vi "setup.vi"(8 "error in (no error)":errorcluster) -> (0 "error out":errorcluster, 3 "DAQmx_pulse_out out":refnum<class "DAQmx_pulse_out.lvclass">)   [LabVIEW 2013, in "DAQmx_pulse_out.lvclass"]
uses:
  DAQmx_pulse_out.lvclass
  DAQmx_pulse_out.lvclass/DAQmx_pulse_out.ctl
  <vilib>/DAQmx/write.llb/DAQmx Write (Digital 1D U8 1Chan NSamp).vi
  Globals.vi
  <vilib>/DAQmx/create/channels.llb/DAQmx Create Channel (DO-Digital Output).vi
  <vilib>/DAQmx/configure/timing.llb/DAQmx Timing (Sample Clock).vi
  <vilib>/DAQmx/configure/trigger.llb/DAQmx Start Trigger (Digital Edge).vi
  <vilib>/DAQmx/miscellaneous.llb/DAQmx Fill In Error Info.vi
panel:
  in  "DAQmx_pulse_out in":refnum<class "DAQmx_pulse_out.lvclass">
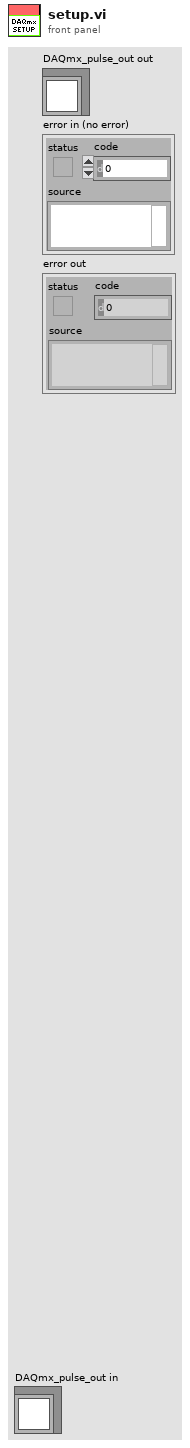
[diagram p1: front panel]
types:
  T1 = typedef "DAQmx_pulse_out.lvclass/settings.ctl" = cluster{"Enable DAQmx Pulses":bool, "DAQmx Physical Channels":tag, "Clock Rate":dbl, "units/sec (ms=1000)":dbl, "Start Trigger":cluster{"Wait for start trigger?":bool, "source":tag, "edge":i32}, "Timing Sequence Control":string[][], "waveform data":u8[]}
  T2 = cluster{"Wait for start trigger?":bool, "source":tag, "edge":i32}
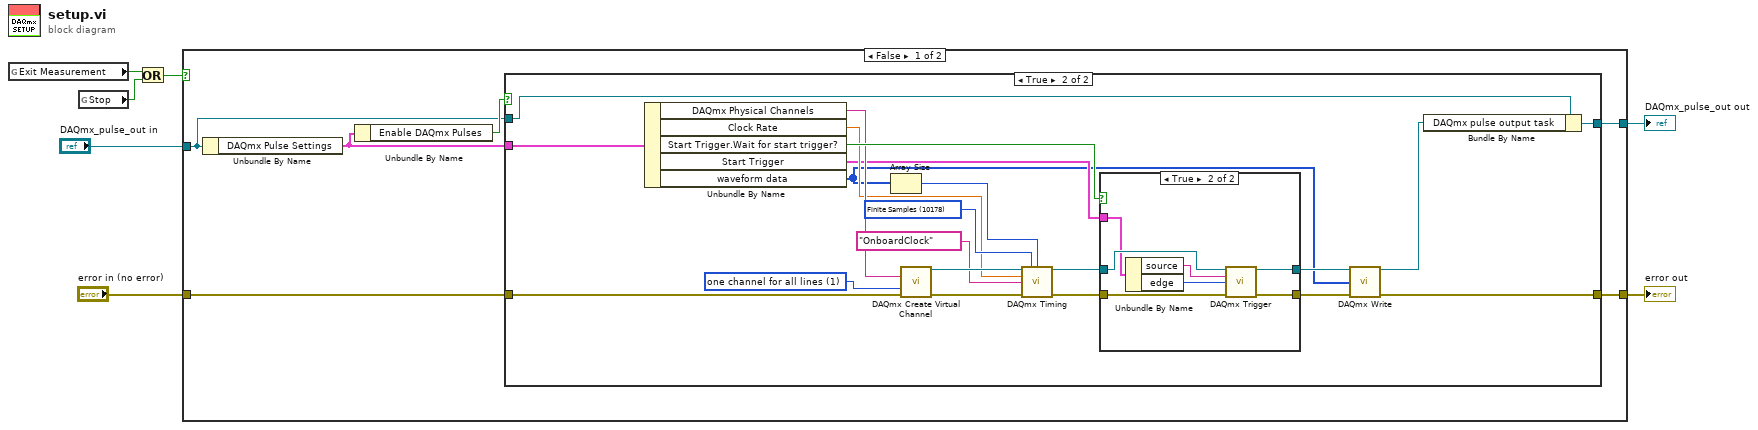
[diagram p0: block diagram]
diagram:
  n1 = global read "Globals.vi" "Exit Measurement"() -> (w3:bool)
  n2 = global read "Globals.vi" "Stop"() -> (w2:bool)
  n3 = Or(x=w3, y=w2) -> (x .or. y?=w1:bool)
  n4 = case shown="False" w1 {
    tunnel: [w12 w46] -> w7
    tunnel: [w13 w47] -> w5
    tunnel: "DAQmx_pulse_out in" -> [w9 w47]
    tunnel: "error in (no error)" -> [w10 w46]
    frame False {
      n5 = Unbundle By Name(w9) -> ("DAQmx Pulse Settings"=w8:T1)
      n6 = Unbundle By Name(w8) -> ("Enable DAQmx Pulses"=w11:bool)
      n7 = case shown="True" w11 {
        tunnel: w10 -> [w14 w20]
        tunnel: w9 -> [w15 w17]
        tunnel: [w15 w32] -> w13
        tunnel: [w14 w31] -> w12
        tunnel: w8 -> [_ w16]
        frame False {
        }
        frame True {
          w23 = 1 items=["one channel for each line", "one channel for all lines"] ("line grouping")
          w34 = 10178 items=["Finite Samples"=10178, "Continuous Samples"=10123, "Hardware Timed Single Point"=12522] ("sample mode")
          n8 = Unbundle By Name(w16) -> ("DAQmx Physical Channels"=w26:tag, "Clock Rate"=w25:dbl, "Start Trigger.Wait for start trigger?"=w27:bool, "Start Trigger"=w24:T2, "waveform data"=w18:u8[])
          n9 = Array Size(array=w18) -> (size(s)=w19:i32)
          n10 = call-poly <vilib>:"DAQmx Create Virtual Channel.vi"("lines"=w26, "line grouping"=w23, "error in"=w20) -> ("task out"=w36:refnum<k21>, "error out"=w35:errorcluster)  [unwired: 11 in]
          n11 = call-poly <vilib>:"DAQmx Timing.vi"("task/channels in"=w36, "sample mode"=w34, "samples per channel"=w19, "rate"=w25, "source"=tag "OnboardClock", "error in"=w35) -> ("task out"=w30:refnum<k21>, "error out"=w28:errorcluster)  [unwired: 8 in]
          n12 = case shown="True" w27 {
            tunnel: w30 -> [w38 w45]
            tunnel: [w38 w44] -> w29
            tunnel: w28 -> [w37 w43]
            tunnel: w24 -> [_ w42]
            tunnel: [w37 w39] -> w22
            frame False {
            }
            frame True {
              n13 = Unbundle By Name(w42) -> ("source"=w41:tag, "edge"=w40:i32)
              n14 = call-poly <vilib>:"DAQmx Trigger.vi"("task/channels in"=w45, "source"=w41, "edge"=w40, "error in"=w43) -> ("task out"=w44:refnum<k21>, "error out"=w39:errorcluster)  [unwired: 10 in]
            }
          }
          n15 = call-poly <vilib>:"DAQmx Write.vi"("task/channels in"=w29, "data"=w18, "error in"=w22) -> ("task out"=w33:refnum<k21>, "error out"=w31:errorcluster)  [unwired: 10 in, 1 out]
          n16 = Bundle By Name(cluster=w17, "DAQmx pulse output task"=w33) -> (w32:refnum<class "DAQmx_pulse_out.lvclass">)
        }
      }
    }
    frame True {
    }
  }
  "error out" <- w7
  "DAQmx_pulse_out out" <- w5
